vi "save i2c.vi"(8 "error in":errorcluster, 10 "path":string, 11 "i2c queue in":refnum<queue>) -> (0 "error out":errorcluster)   [LabVIEW 2025, in "Automotive Vision.lvclass"]
uses:
  Automotive Vision.lvclass
  Automotive Vision.lvclass/Automotive Vision.ctl
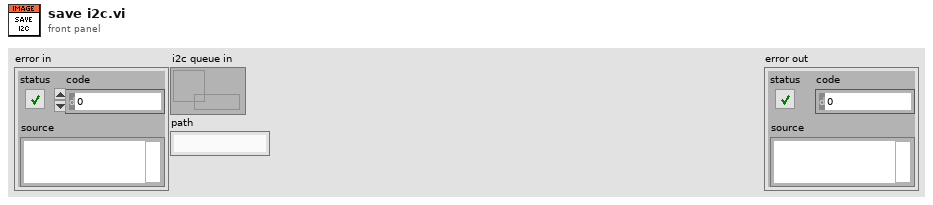
[diagram p1: front panel]
types:
  T1 = enum16{"open", "replace", "create", "open or create", "replace or create", "replace or create with confirmation"}
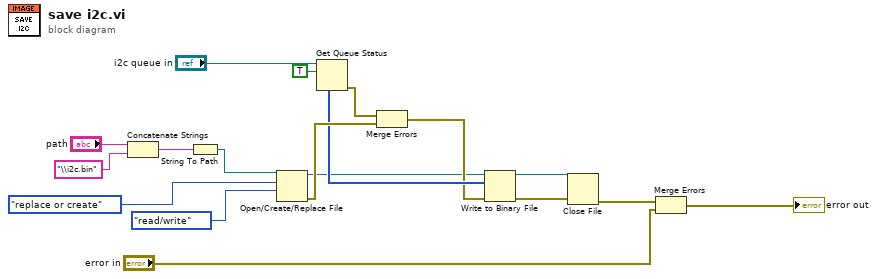
[diagram p0: block diagram]
diagram:
  n1 = Concatenate Strings("path", "\\i2c.bin" ("element")) -> (w2:string)
  n2 = String To Path(string=w2) -> (path=w1:path)
  n3 = Open/Create/Replace File(file path (use dialog)=w1, operation (0:open)=T1."replace or create", access (0:read/write)=enum16{"read/write", "read-only", "write-only"}."read/write") -> (refnum out=w10:refnum<file>, error out=w13:errorcluster)  [unwired: 3 in, 1 out]
  n4 = Get Queue Status(queue="i2c queue in", return elements? (F)=TRUE) -> (error out=w14:errorcluster, elements=w12:u64[])  [unwired: 1 in, 6 out]
  n5 = Merge Errors(w14, w13) -> (w11:errorcluster)
  n6 = Write to Binary File(file (use dialog)=w10, data=w12, error in=w11) -> (refnum out=w8:refnum<file>, error out=w9:errorcluster)  [unwired: 3 in, 1 out]
  n7 = Close File(refnum=w8, error in=w9) -> (error out=w6:errorcluster)  [unwired: 1 out]
  n8 = Merge Errors(w6, "error in") -> (→"error out":errorcluster)
